vi "ConfigInstr.vi"(6 "InstrumentName":string, 7 "VisaRessIn":refnum<visa-resource-name>, 8 "error in (no error)":errorcluster caption="entrée d'erreur (pas d'erreur)", 9 "FirstClassInst":bool, 10 "Function":string, 11 "GenData In":refnum<class "KlingerMotor.lvclass"> caption="DNL_LabVIEW Object in") -> (0 "error out":errorcluster caption="sortie d'erreur", 3 "GenData Out":refnum<class "KlingerMotor.lvclass"> caption="DNL_LabVIEW Object out")   [LabVIEW 2019, in "KlingerMotor.lvclass"]
uses:
  KlingerMotor.lvclass
  C:/Programmes Labview/LabScanV1A/DevicesClass/BaseDevice/BaseDevice.lvclass
  KlingerMotor_Func.ctl
  KlingerMotor.lvclass/KlingerMotor.ctl
  <userlib>/KlingerV2/KlingerV2 Params.ctl
  BaseDevice/BaseDevice.lvclass/BaseDevice.ctl
  BaseDevice/Accessor/SetShowInstrNm.vi
  BaseDevice/Accessor/SetScanPanelPath.vi
  BaseDevice/Accessor/SetInstrParam.vi
panel:
  in  "Class_Func":T1
  out "VisaRessOut":refnum<visa-resource-name>
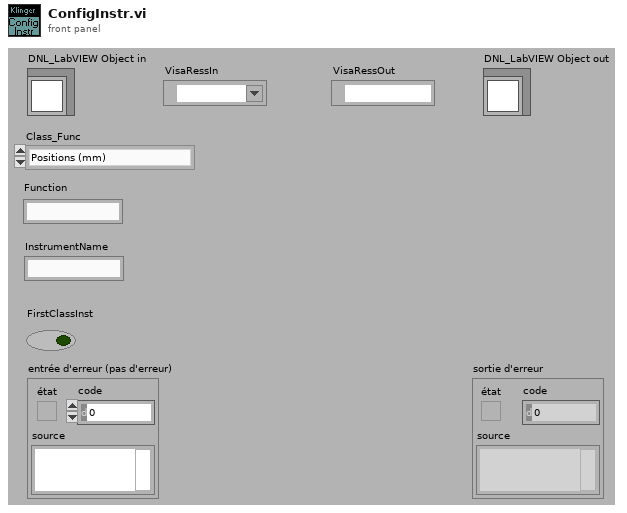
[diagram p1: front panel]
types:
  T1 = typedef "KlingerMotor.lvclass/KlingerMotor_Func.ctl" = enum16{"Positions (mm)", "Position (deg)", "PositionWithTrig (deg)", "Position (ps)", "ReadWPos (ps)", "ReadWPos (mm)", "ReadZPos (ps)", "ReadZPos (mm)", "DOTrigger (Point)"}
  T2 = typedef "KlingerV2 Params.ctl" = enum16{"Type", "Origine", "Encodeur", "TypeMouv", "FactConv", "Nom", "CorrParams", "KlingCtrlPar", "Speed", "Acc", "Avance", "Tous"}
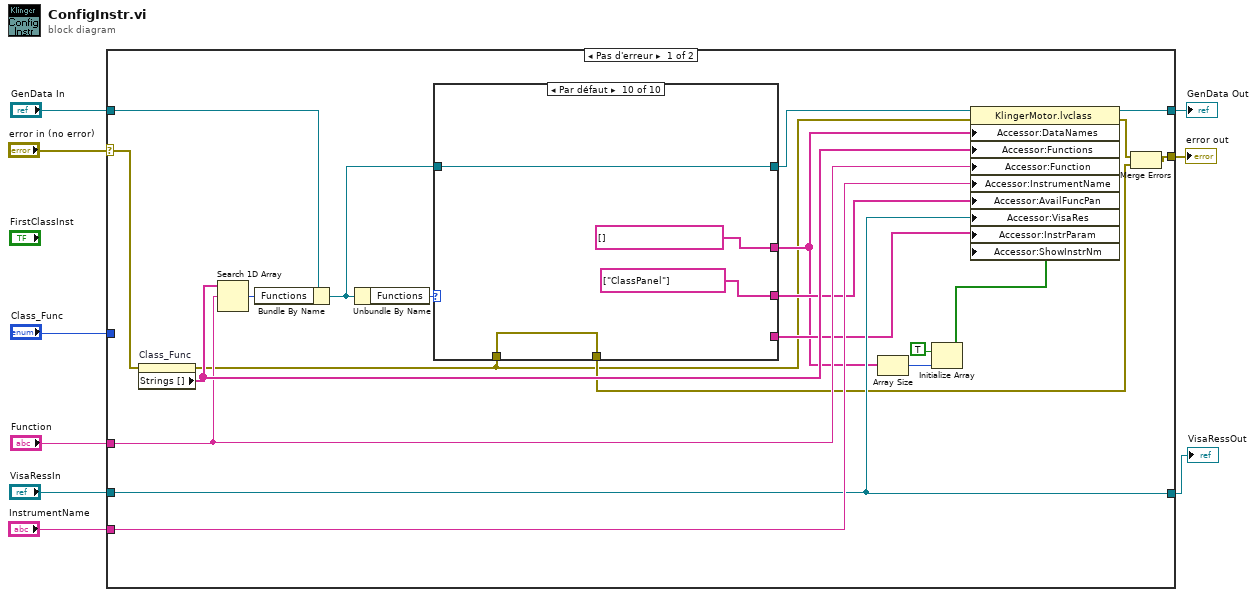
[diagram p0: block diagram]
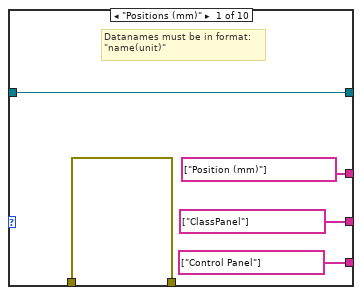
[diagram p2: hidden frame]
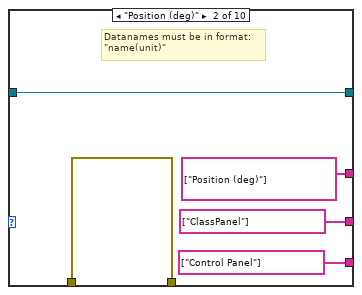
[diagram p3: hidden frame]
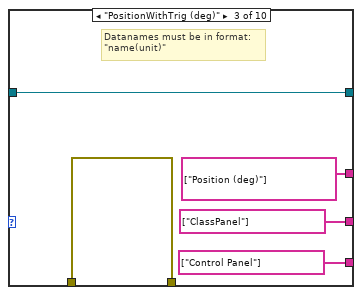
[diagram p4: hidden frame]
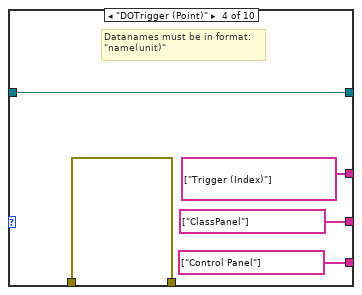
[diagram p5: hidden frame]
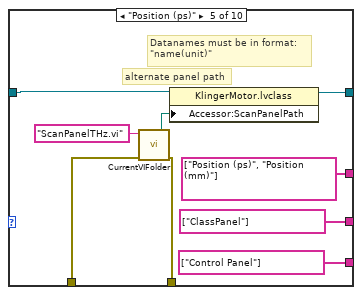
[diagram p6: hidden frame]
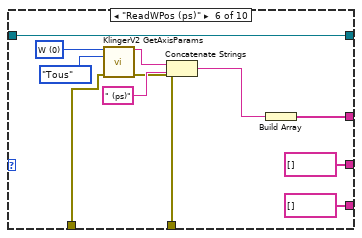
[diagram p7: hidden frame]
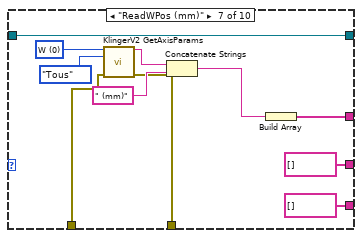
[diagram p8: hidden frame]
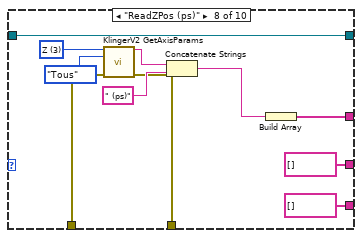
[diagram p9: hidden frame]
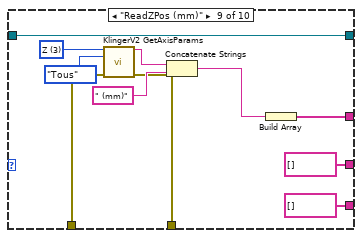
[diagram p10: hidden frame]
diagram:
  n1 = case shown="Pas d'erreur" "error in (no error)" {
    selector: "error in (no error)" -> [w24 w109]
    tunnel: [w12 w109] -> w8
    tunnel: "GenData In" -> [w25 w108]
    tunnel: [w29 w108] -> w6
    tunnel: "Class_Func" -> [_ _]
    tunnel: "Function" -> [w21 _]
    tunnel: "InstrumentName" -> [w20 _]
    tunnel: "VisaRessIn" -> [w18 _]
    tunnel: [w18 _] -> w1
    frame No Error {
      n2 = property on="Class_Func" class="Énum (strict)"(error in=w24) -> (error out=w10:errorcluster, "Strings []"=w27:string[])  [unwired: 1 in, 1 out]
      n3 = Search 1D Array(1D array=w27, element=w21) -> (index of element=w26:i32)  [unwired: 1 in]
      n4 = Bundle By Name(cluster=w25, "Functions"=w26) -> (w23:refnum<class "KlingerMotor.lvclass">)
      n5 = Unbundle By Name(w23) -> ("Functions"=w28:T1)
      n6 = case shown="Par défaut" w28 {
        tunnel: [string[] ["Position (mm)"] string[] ["Position (deg)"] string[] ["Position (deg)"] string[] ["Trigger (Index)"] string[] ["Position (ps)", "Position (mm)"] w62 w73 w84 w95 string[] []] -> w14
        tunnel: w23 -> [w32 w36 w42 w47 w59 w68 w79 w90 w101 w106]
        tunnel: [w32 w36 w42 w47 w55 w68 w79 w90 w101 w106] -> w22
        tunnel: [string[] ["ClassPanel"] string[] ["ClassPanel"] string[] ["ClassPanel"] string[] ["ClassPanel"] string[] ["ClassPanel"] string[] [] string[] [] string[] [] string[] [] string[] ["ClassPanel"]] -> w19
        tunnel: [string[] ["Control Panel"] string[] ["Control Panel"] string[] ["Control Panel"] string[] ["Control Panel"] string[] ["Control Panel"] string[] [] string[] [] string[] [] string[] [] _] -> w17
        tunnel: [w31 w37 w41 w46 w51 w60 w71 w83 w94 w104] -> w11
        tunnel: w10 -> [w31 w37 w41 w46 w52 w61 w72 w82 w93 w104]
        frame "Positions (mm)" {
          # "Datanames must be in format:\n\"name(unit)\""
        }
        frame "Position (deg)" {
          # "Datanames must be in format:\n\"name(unit)\""
        }
        frame "PositionWithTrig (deg)" {
          # "Datanames must be in format:\n\"name(unit)\""
        }
        frame "DOTrigger (Point)" {
          # "Datanames must be in format:\n\"name(unit)\""
        }
        frame "Position (ps)" {
          # "alternate panel path"
          # "Datanames must be in format:\n\"name(unit)\""
          n7 = call <userlib>:"CurrentVIFolder.vi"("error in (no error)"=w52, "NomFichier"="ScanPanelTHz.vi") -> ("error out"=w51:errorcluster, "Chemin"=w54:path)  [unwired: 7 in, 1 out]
          n8 = property class="KlingerMotor.lvclass"(reference=w59, "Accessor:ScanPanelPath"=w54) -> (reference out=w55:refnum<class "KlingerMotor.lvclass">)  [unwired: 1 in, 1 out]
        }
        frame "ReadWPos (ps)" {
          w67 = u8 0 items=["W", "X", "Y", "Z"] ("Axe")
          n9 = call <userlib>:"KlingerV2 GetAxisParams.vi"("Axe"=w67, "Param"=KlingerV2_Params."Tous", "error in"=w61) -> ("Nom de l'axe"=w65:string, "error out"=w60:errorcluster)  [unwired: 3 in, 8 out]
          n10 = Concatenate Strings(w65, " (ps)" ("string")) -> (w63:string)
          n11 = Build Array(w63) -> (w62:string[])
        }
        frame "ReadWPos (mm)" {
          w78 = u8 0 items=["W", "X", "Y", "Z"] ("Axe")
          n12 = call <userlib>:"KlingerV2 GetAxisParams.vi"("Axe"=w78, "Param"=KlingerV2_Params."Tous", "error in"=w72) -> ("Nom de l'axe"=w76:string, "error out"=w71:errorcluster)  [unwired: 3 in, 8 out]
          n13 = Concatenate Strings(w76, " (mm)" ("string")) -> (w74:string)
          n14 = Build Array(w74) -> (w73:string[])
        }
        frame "ReadZPos (ps)" {
          w89 = u8 3 items=["W", "X", "Y", "Z"] ("Axe")
          n15 = call <userlib>:"KlingerV2 GetAxisParams.vi"("Axe"=w89, "Param"=KlingerV2_Params."Tous", "error in"=w82) -> ("Nom de l'axe"=w87:string, "error out"=w83:errorcluster)  [unwired: 3 in, 8 out]
          n16 = Concatenate Strings(w87, " (ps)" ("string")) -> (w85:string)
          n17 = Build Array(w85) -> (w84:string[])
        }
        frame "ReadZPos (mm)" {
          w100 = u8 3 items=["W", "X", "Y", "Z"] ("Axe")
          n18 = call <userlib>:"KlingerV2 GetAxisParams.vi"("Axe"=w100, "Param"=KlingerV2_Params."Tous", "error in"=w93) -> ("Nom de l'axe"=w98:string, "error out"=w94:errorcluster)  [unwired: 3 in, 8 out]
          n19 = Concatenate Strings(w98, " (mm)" ("string")) -> (w96:string)
          n20 = Build Array(w96) -> (w95:string[])
        }
        frame Default {
        }
      }
      n21 = Array Size(array=w14) -> (size(s)=w16:i32)
      n22 = Initialize Array(TRUE, w16) -> (w13:bool[])
      n23 = property class="KlingerMotor.lvclass"(reference=w22, error in=w10, "Accessor:DataNames"=w14, "Accessor:Functions"=w27, "Accessor:Function"=w21, "Accessor:InstrumentName"=w20, "Accessor:AvailFuncPan"=w19, "Accessor:VisaRes"=w18, "Accessor:InstrParam"=w17, "Accessor:ShowInstrNm"=w13) -> (reference out=w29:refnum<class "KlingerMotor.lvclass">, error out=w30:errorcluster)
      n24 = Merge Errors(w30, w11) -> (w12:errorcluster)
    }
    frame Error {
    }
  }
  "error out" <- w8
  "GenData Out" <- w6
  "VisaRessOut" <- w1
